vi "UpdateSaveData.vi"(1 "ModelEditInfo in":T1) -> (0 "ModelEditInfo out":T1)   [LabVIEW 2014]
uses:
  <vilib>/Utility/file.llb/Write To Spreadsheet File (string).vi
  ModeEditeControl.ctl
  ModelInfo.ctl
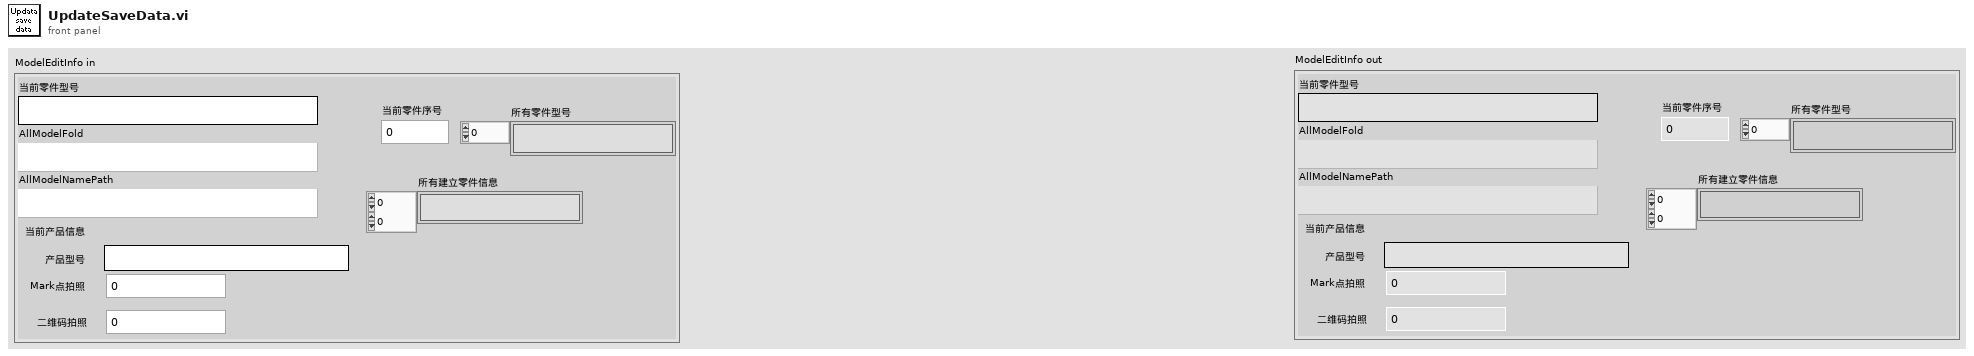
[diagram p1: front panel]
types:
  T1 = typedef "ModeEditeControl.ctl" = cluster{"AllModelFold":path, "AllModelNamePath":path, "所有零件型号":string[], "当前零件型号":string, "所有建立零件信息":string[][], "当前零件序号":i32, "当前产品信息":T2}
  T2 = typedef "ModelInfo.ctl" = cluster{"产品型号":string, "二维码拍照":u32, "Mark点拍照":u32}
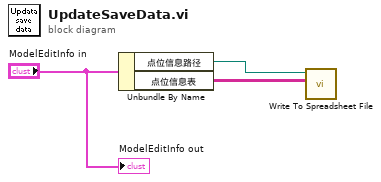
[diagram p0: block diagram]
diagram:
  n1 = Unbundle By Name("ModelEditInfo in") -> ("点位信息路径"=w2:path, "点位信息表"=w1:string[][])
  n2 = call-poly <vilib>:"Write To Spreadsheet File.vi"("2D data"=w1, "file path (dialog if empty)"=w2) -> ()  [unwired: 6 in, 1 out]
  "ModelEditInfo out" <- "ModelEditInfo in"
